vi "bk9201 Set.vi"(6 "Enable Output":bool, 9 "Current":dbl format="%.2f", 10 "Voltage":dbl format="%.2g", 11 "VISA resource name":refnum<visa-resource-name>="USB0::0xFFFF::0x9200::802243020766810010::INSTR") -> (0 "error out":errorcluster)   [LabVIEW 2018]
uses:
  <instrlib>/BK Precision 9200 Series/BK Precision 9200 Series.lvlib
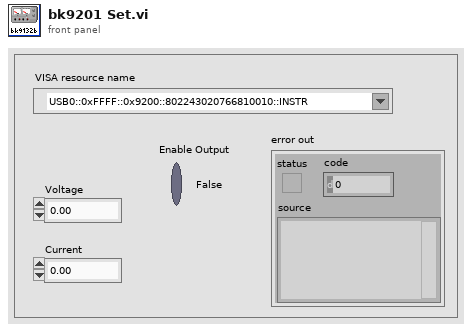
[diagram p1: front panel]
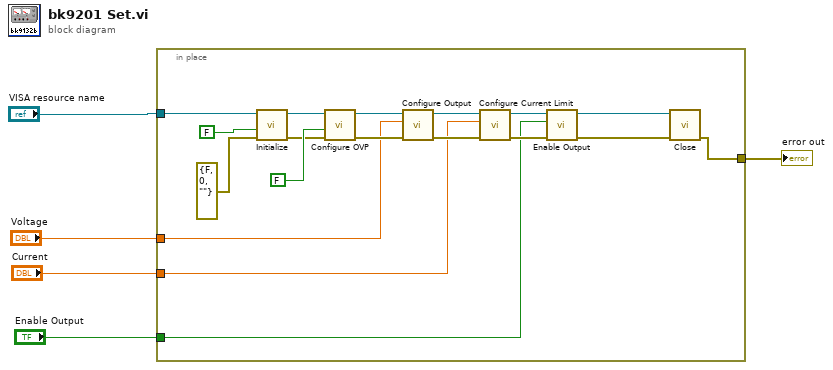
[diagram p0: block diagram]
diagram:
  n1 = in-place {
    in-place-border: "VISA resource name" -> [w22]
    in-place-border: [w21] -> w4
    in-place-border: "Voltage" -> [w14]
    in-place-border: "Current" -> [w11]
    in-place-border: "Enable Output" -> [w6]
    n2 = call <instrlib>:"Initialize.vi"("error in (no error)"=errorcluster {"status"=FALSE, "code"=0, "source"=""}, "Reset (True)"=FALSE, "VISA resource name"=w22) -> ("error out"=w17:errorcluster, "VISA resource name out"=w18:refnum<visa-resource-name>)  [unwired: 7 in]
    n3 = call <instrlib>:"Configure OVP.vi"("error in (no error)"=w17, "Enable OVP (T: Enable)"=FALSE, "VISA resource name"=w18) -> ("error out"=w15:errorcluster, "VISA resource name out"=w16:refnum<visa-resource-name>)  [unwired: 7 in]
    n4 = call <instrlib>:"Configure Output.vi"("error in (no error)"=w15, "Voltage Level (0.0 V)"=w14, "VISA resource name"=w16) -> ("error out"=w12:errorcluster, "VISA resource name out"=w13:refnum<visa-resource-name>)  [unwired: 7 in]
    n5 = call <instrlib>:"Configure Current Limit.vi"("error in (no error)"=w12, "Current Limit (0.0 A)"=w11, "VISA resource name"=w13) -> ("error out"=w10:errorcluster, "VISA resource name out"=w7:refnum<visa-resource-name>)  [unwired: 7 in]
    n6 = call <instrlib>:"Enable Output.vi"("error in (no error)"=w10, "Enable Output (F: False)"=w6, "VISA resource name"=w7) -> ("error out"=w9:errorcluster, "VISA resource name out"=w8:refnum<visa-resource-name>)  [unwired: 7 in]
    n7 = call <instrlib>:"Close.vi"("error in (no error)"=w9, "VISA resource name"=w8) -> ("error out"=w21:errorcluster)  [unwired: 9 in]
  }
  "error out" <- w4
